vi "Test Method Not Dashed.vi"(8 "error in (no error)":errorcluster, 11 "Dummy Test Case in":refnum<class "_Dashed Library Dummy.lvclass">) -> (0 "error out":errorcluster, 3 "Dummy Test Case out":refnum<class "_Dashed Library Dummy.lvclass">)   [LabVIEW 2020, in "Test Library.lvlib" / "_Dashed Library Dummy.lvclass"]
uses:
  _Dashed Library Dummy.lvclass
  _Dashed Library Dummy.lvclass/_Dashed Library Dummy.ctl
  source/API/LUnit Test Case/LUnit Test Case.lvclass
  C:/git/astemes-lunit/source/API/LUnit Test Case/LUnit Test Case.lvclass
  C:/git/astemes-lunit/source/Core/Runnable/Runnable.lvclass
  C:/git/astemes-lunit/tests/Filter Test/Dashed Dummy in Library/_Dashed Library Dummy.lvclass
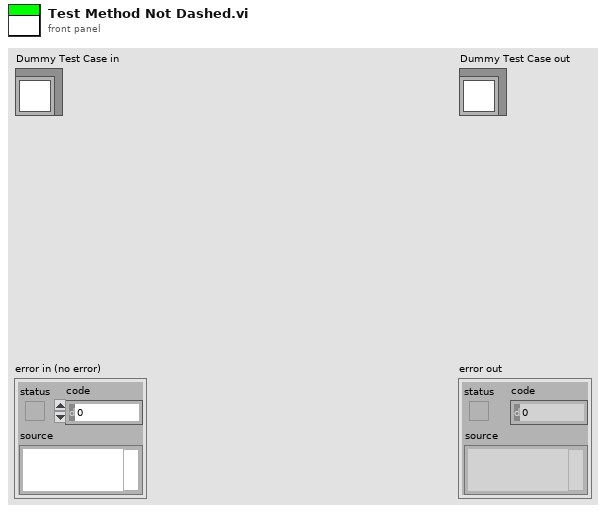
[diagram p1: front panel]
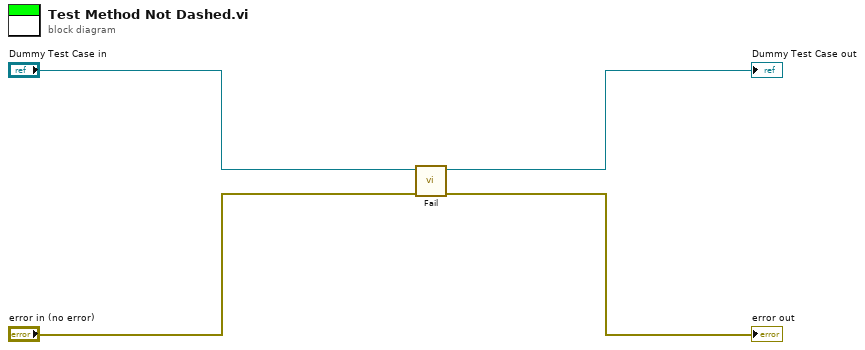
[diagram p0: block diagram]
diagram:
  n1 = call "Fail.vi"("error in (no error)"="error in (no error)", "LUnit Test Case In"="Dummy Test Case in") -> ("error out"=→"error out":errorcluster, "LUnit Test Case Out"=→"Dummy Test Case out":refnum<class "_Dashed Library Dummy.lvclass">)  [unwired: 8 in]
